vi "statistics.vi"(11 "Wash Log Path":refnum<vi>) -> (1 "Wash Graph":refnum<class "3D Plot Datatype.lvclass">[](xcontrol), 2 "sum-ew":dbl caption="Total Economy Wash", 3 "sum-dw":dbl caption="Total Deluxe Wash", 4 "All Wash Data":string[][](array[string]))   [LabVIEW 2021]
uses:
  <vilib>/Math Plots/3D Math Plots/3D Bar/3D Bar XCtrl/3D Bar.xctl
  <vilib>/Utility/file.llb/Read Delimited Spreadsheet (string).vi
  <vilib>/Math Plots/3D Math Plots/3D Bar/3D Bar Datatype/Public/Plot Helper (Matrix).vi
  <vilib>/Math Plots/3D Math Plots/3D Bar/3D Bar Datatype/3D Bar Datatype.lvclass
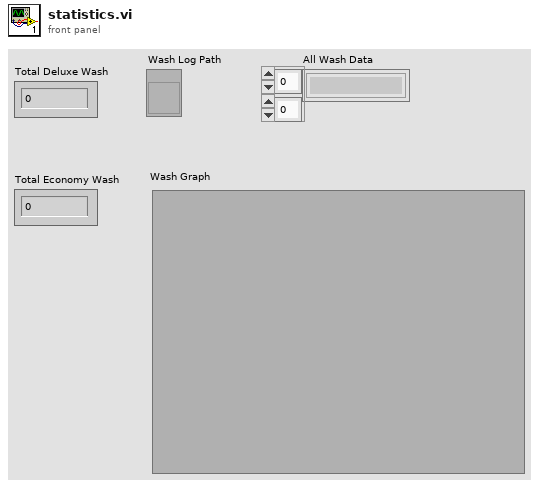
[diagram p1: front panel]
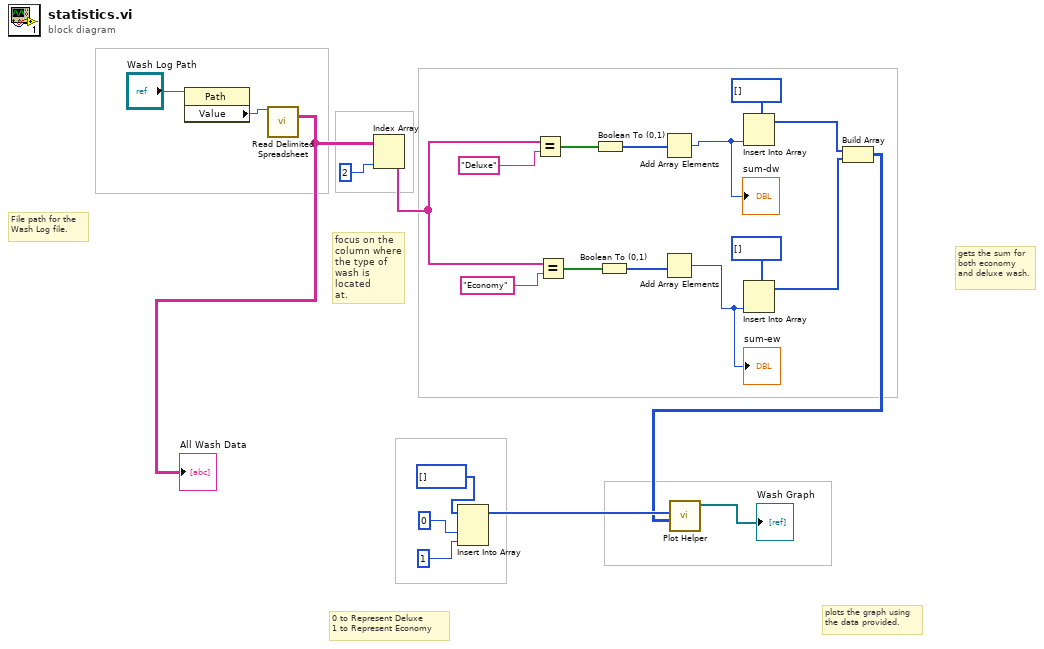
[diagram p0: block diagram]
diagram:
  # "0 to Represent Deluxe\n1 to Represent Economy"
  # "File path for the\nWash Log file."
  # "focus on the\ncolumn where\nthe type of\nwash is located\nat."
  # "gets the sum for\nboth economy\nand deluxe wash."
  # "plots the graph using\nthe data provided."
  n1 = property class="Path"(reference="Wash Log Path") -> ("Value"=w2:path)  [unwired: 1 in, 2 out]
  n2 = call-poly <vilib>:"Read Delimited Spreadsheet.vi"("file path (dialog if empty)"=w2) -> ("all rows"=w4:string[][])  [unwired: 9 in, 5 out]
  "All Wash Data" <- w4
  n3 = Index Array "Index Array"(array=w4, index (col)=2 ("disabled index (col)")) -> (element=w5:string[])  [unwired: 1 in]
  n4 = Insert Into Array(array=i16[] [], new element #1=i16 0 ("new element/subarray"), new element #2=i16 1 ("new element/subarray")) -> (w23:i16[])  [unwired: 1 in]
  n5 = Equal?(x=w5, y="Deluxe") -> (x = y?=w8:bool[])
  n6 = Equal?(x=w5, y="Economy") -> (x = y?=w9:bool[])
  n7 = Boolean To (0,1)(Boolean=w8) -> (0, 1=w10:i16[])
  n8 = Boolean To (0,1)(Boolean=w9) -> (0, 1=w11:i16[])
  n9 = Add Array Elements(numeric array=w10) -> (sum=w20:i16)
  "sum-dw" <- w20
  n10 = Add Array Elements(numeric array=w11) -> (sum=w21:i16)
  "sum-ew" <- w21
  n11 = Insert Into Array(array=i16[] [], new element=w20) -> (w17:i16[])  [unwired: 1 in]
  n12 = Insert Into Array(array=i16[] [], new element=w21) -> (w18:i16[])  [unwired: 1 in]
  n13 = Build Array(w17, w18) -> (w22:i16[][])
  n14 = call-poly <vilib>:"Plot Helper.vi"("z matrix"=w22, "y vector"=w23) -> ("3D Plot lvclass Array out"=→"Wash Graph":refnum<class "3D Plot Datatype.lvclass">[])  [unwired: 1 in, 8 out]
